vi "GetImageSize.vi"(8 "error in (no error)":errorcluster, 11 "Camera in":refnum<class "Camera.lvclass">) -> (0 "error out":errorcluster, 1 "ImageSize(Mb)":dbl, 2 "ImageSize(Kb)":dbl, 3 "Camera out":refnum<class "Camera.lvclass">)   [LabVIEW 2020, in "Camera.lvlib" / "Camera.lvclass"]
uses:
  Camera.lvclass
  Camera.lvclass/Camera.ctl
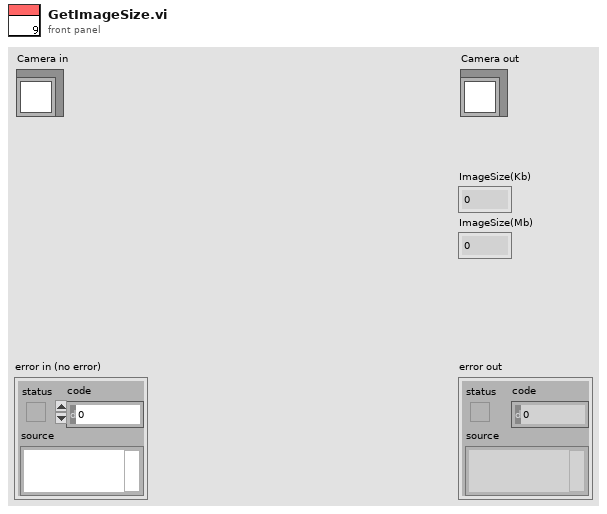
[diagram p1: front panel]
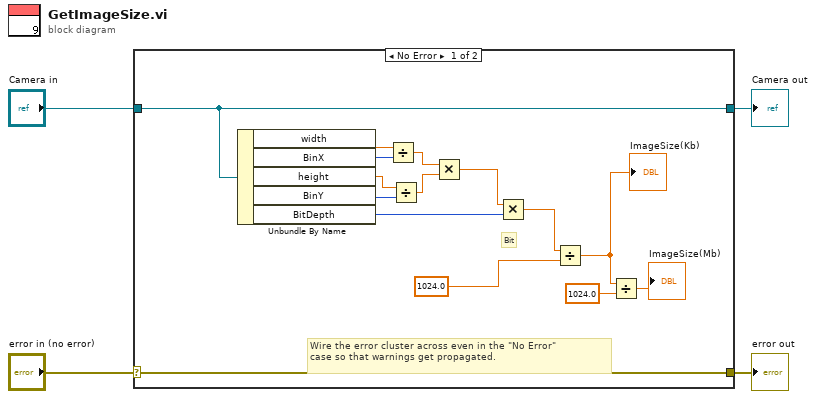
[diagram p0: block diagram]
diagram:
  n1 = case shown="No Error" "error in (no error)" {
    selector: "error in (no error)" -> [w19 w21]
    tunnel: [w19 w21] -> w3
    tunnel: [w18 w20] -> w1
    tunnel: "Camera in" -> [w18 w20]
    frame No Error {
      # "Bit"
      # "Wire the error cluster across even in the \"No Error\"\ncase so that warnings get propagated."
      n2 = Unbundle By Name(w18) -> ("width"=w17:dbl, "BinX"=w16:i32, "height"=w15:dbl, "BinY"=w14:i32, "BitDepth"=w11:i32)
      n3 = Divide(x=w17, y=w16) -> (x/y=w13:dbl)
      n4 = Divide(x=w15, y=w14) -> (x/y=w12:dbl)
      n5 = Multiply(x=w13, y=w12) -> (x*y=w10:dbl)
      n6 = Multiply(x=w10, y=w11) -> (x*y=w9:dbl)
      n7 = Divide(x=w9, y=1024.0) -> (x/y=w7:dbl)
      "ImageSize(Kb)" <- w7
      n8 = Divide(x=w7, y=1024.0) -> (x/y=→"ImageSize(Mb)":dbl)
    }
    frame Error {
    }
  }
  "error out" <- w3
  "Camera out" <- w1
